vi "draw.vi"(0 "reference":refnum<class "RectangularNode.lvclass">, 1 "graphics":refnum<class "Graphics.lvclass">, 5 "error in (no error)":errorcluster) -> (14 "reference out":refnum<class "RectangularNode.lvclass">, 19 "error out":errorcluster)   [LabVIEW 2016, in "RectangularNode.lvclass"]
doc: "public void draw(Graphics2D g2, Point2D p, Point2D q)"
uses:
  <resource>/Framework/Providers/Open_GDS/UML/RectangularNode_class/RectangularNode.lvclass
  <resource>/Framework/Providers/Open_GDS/UML/Graphics_class/Graphics.lvclass
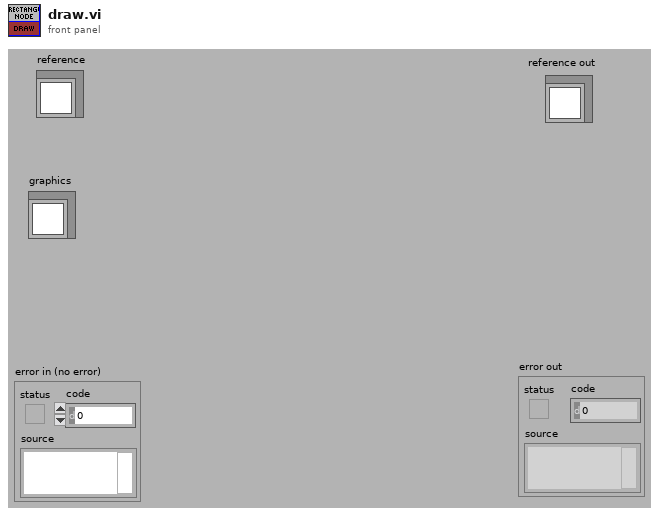
[diagram p1: front panel]
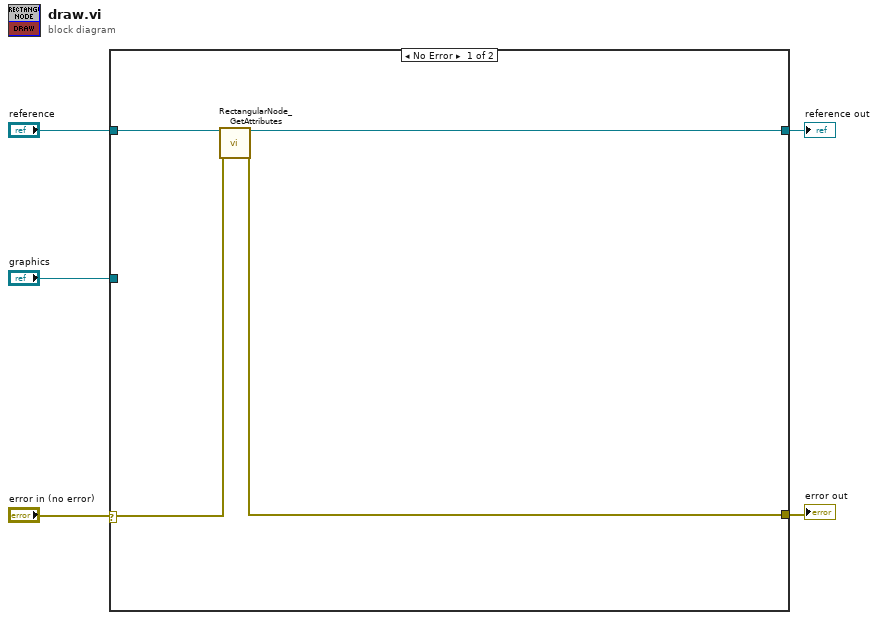
[diagram p0: block diagram]
diagram:
  n1 = case shown="No Error" "error in (no error)" {
    selector: "error in (no error)" -> [w6 w10]
    tunnel: "reference" -> [w9 w11]
    tunnel: [w8 w10] -> w4
    tunnel: [w7 w11] -> w3
    tunnel: "graphics" -> [_ _]
    frame No Error {
      n2 = call <resource>:"RectangularNode_GetAttributes.vi"("reference in"=w9, "error in (no error)"=w6) -> ("reference out"=w7:refnum<class "RectangularNode.lvclass">, "error out"=w8:errorcluster)  [unwired: 1 in, 15 out]
    }
    frame Error {
    }
  }
  "reference out" <- w3
  "error out" <- w4
